vi "28_Image Animations.vi"() -> ()   [LabVIEW 2022 SP3]
panel:
  in  "stop":bool
  in  "Knob":dbl(knob) scale=0.0..200.0
  out "Bird Movie":u16(ring)
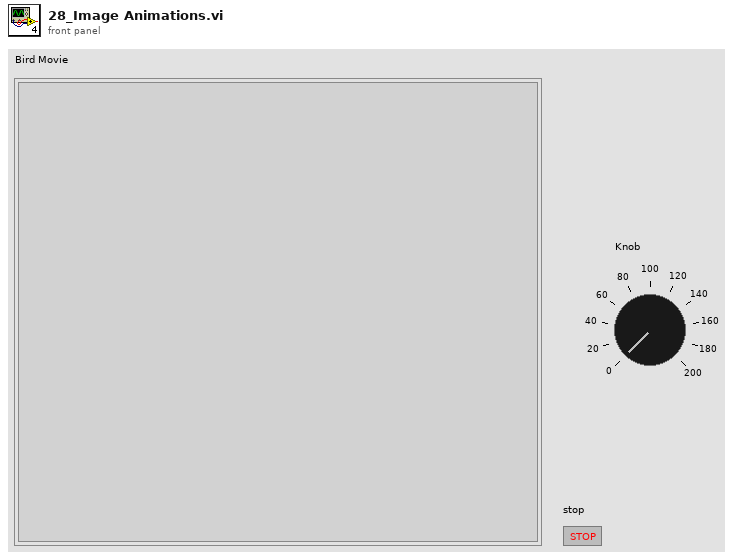
[diagram p1: front panel]
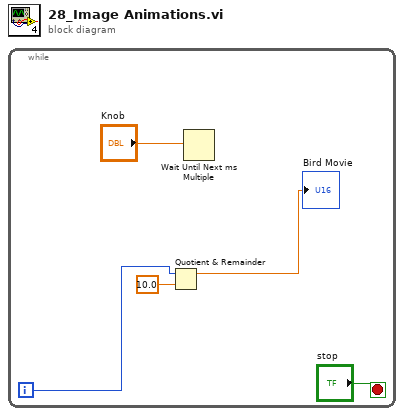
[diagram p0: block diagram]
diagram:
  n1 = while {
    i -> [w3]
    stop <- "stop" stop-if-true
    n2 = Quotient & Remainder(x=w3, y=10.0) -> (x-y*floor(x/y)=→"Bird Movie":dbl)  [unwired: 1 out]
    n3 = Wait Until Next ms Multiple(millisecond multiple="Knob") -> ()  [unwired: 1 out]
  }
